vi "Pre.vi"(8 "Error In":errorcluster, 11 "Compile In":refnum<class "Mock Compile Hook.lvclass">) -> (0 "Error Out":errorcluster, 3 "Compile Out":refnum<class "Mock Compile Hook.lvclass">)   [LabVIEW 2018, in "Tests.lvlib" / "Compile.lvlib" / "Mock Compile Hook.lvclass"]
uses:
  Mock Compile Hook.lvclass
  Mock Compile Hook.lvclass/Mock Compile Hook.ctl
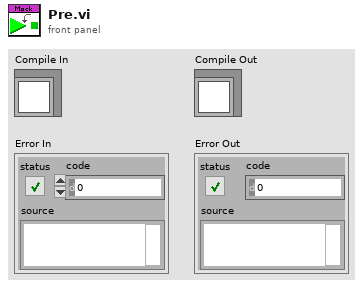
[diagram p1: front panel]
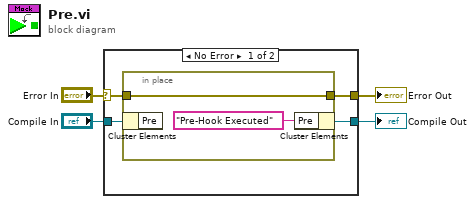
[diagram p0: block diagram]
diagram:
  n1 = case shown="No Error" "Error In" {
    selector: "Error In" -> [w6 w12]
    tunnel: [w5 w12] -> w3
    tunnel: "Compile In" -> [w8 w11]
    tunnel: [w7 w11] -> w1
    frame No Error {
      n2 = in-place {
        in-place-border: w6 -> [w9]
        in-place-border: [w9] -> w5
        n3 = in-place-cluster #1(w8) -> ()  [unwired: 1 out]
        n4 = in-place-cluster #1("Pre"="Pre-Hook Executed") -> (w7:refnum<class "Mock Compile Hook.lvclass">)
      }
    }
    frame Error {
    }
  }
  "Compile Out" <- w1
  "Error Out" <- w3
